vi "Day 2.1 - Calculate postion.vi"(11 "input":string[](array[string])) -> (3 "output":i32)   [LabVIEW 2021]
uses:
  Controls/submarine position.ctl
panel:
  out "submarine position":T1
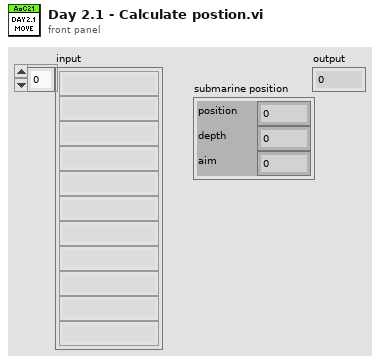
[diagram p1: front panel]
types:
  T1 = typedef "submarine position.ctl" = cluster{"position":i32, "depth":i32, "aim":i32}
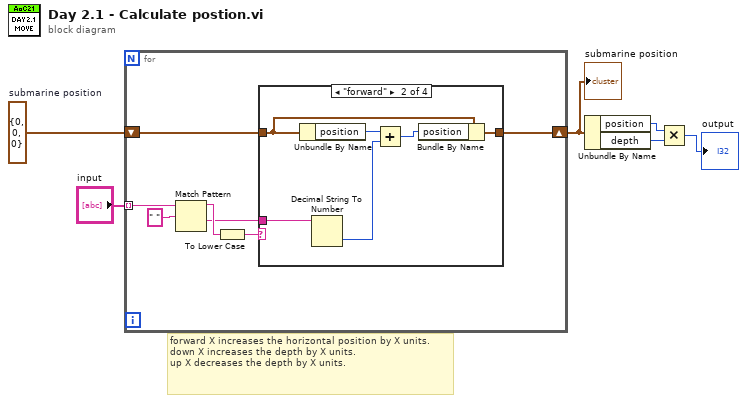
[diagram p0: block diagram]
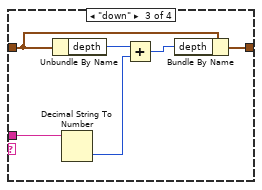
[diagram p3: hidden frame]
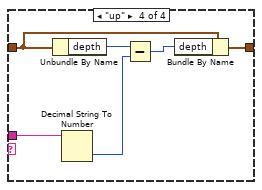
[diagram p4: hidden frame]
diagram:
  w5 = T1 {"position"=0, "depth"=0, "aim"=0}  # submarine position
  # "forward X increases the horizontal position by X units.\ndown X increases the depth by X units.\nup X decreases the depth by X units."
  n1 = for {
    tunnel: "input" -> [w11] mode=indexing
    shift-right: [w12] -> w4
    shift-left: w5 -> [w13]
    n2 = Match Pattern(string=w11, regular expression=" ") -> (before substring=w9:string, after substring=w7:string)  [unwired: 1 in, 2 out]
    n3 = To Lower Case(string=w9) -> (all lower case string=w8:string)
    n4 = case shown="\"forward\"" w8 {
      tunnel: w13 -> [w14 w15 w21 w27]
      tunnel: [w14 w16 w22 w28] -> w12
      tunnel: w7 -> [_ w20 w26 w32]
      frame Default {
      }
      frame "forward" {
        n5 = Unbundle By Name(w15) -> ("position"=w18:i32)
        n6 = Decimal String To Number(string=w20) -> (number=w19:i32)  [unwired: 2 in, 1 out]
        n7 = Add(x=w18, y=w19) -> (x+y=w17:i32)
        n8 = Bundle By Name(cluster=w15, "position"=w17) -> (w16:T1)
      }
      frame "down" {
        n9 = Unbundle By Name(w21) -> ("depth"=w24:i32)
        n10 = Decimal String To Number(string=w26) -> (number=w25:i32)  [unwired: 2 in, 1 out]
        n11 = Add(x=w24, y=w25) -> (x+y=w23:i32)
        n12 = Bundle By Name(cluster=w21, "depth"=w23) -> (w22:T1)
      }
      frame "up" {
        n13 = Unbundle By Name(w27) -> ("depth"=w30:i32)
        n14 = Decimal String To Number(string=w32) -> (number=w31:i32)  [unwired: 2 in, 1 out]
        n15 = Subtract(x=w30, y=w31) -> (x-y=w29:i32)
        n16 = Bundle By Name(cluster=w27, "depth"=w29) -> (w28:T1)
      }
    }
  }
  "submarine position" <- w4
  n17 = Unbundle By Name(w4) -> ("position"=w3:i32, "depth"=w2:i32)
  n18 = Multiply(x=w3, y=w2) -> (x*y=→"output":i32)
